vi "Calculate Progress.vi"(0 "Total Iterations":i32, 1 "Current Iteration":i32) -> (14 "Progress":u8)   [LabVIEW 2010, in "TDMS to ASCII Convert.lvlib"]
uses:
  TDMS to ASCII Convert.lvlib
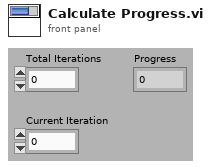
[diagram p1: front panel]
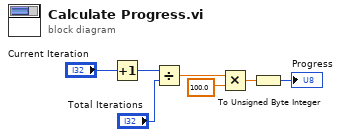
[diagram p0: block diagram]
diagram:
  n1 = Increment(x="Current Iteration") -> (x+1=w2:i32)
  n2 = Divide(x=w2, y="Total Iterations") -> (x/y=w5:dbl)
  n3 = Multiply(x=w5, y=100.0) -> (x*y=w3:dbl)
  n4 = To Unsigned Byte Integer(number=w3) -> (unsigned 8bit integer=→"Progress":u8)
